vi "set_xwav_attribute_by_name.vi"(8 "Error in":errorcluster caption="Error in (no error)", 9 "value":variant, 10 "name":string, 11 "xwave in":T1={"attributes"=variant, "X"={"start"=0.0, "delta"=0.0, "units"="index", "dim"="au"}, "Y"={"data"=[], "units"="au"}}) -> (0 "Error out":errorcluster, 2 "replaced?":bool, 3 "xwave out":T1={"attributes"=variant, "X"={"start"=0.0, "delta"=0.0, "units"="index", "dim"="au"}, "Y"={"data"=[], "units"="au"}})   [LabVIEW 2015]
uses:
  xwav.ctl
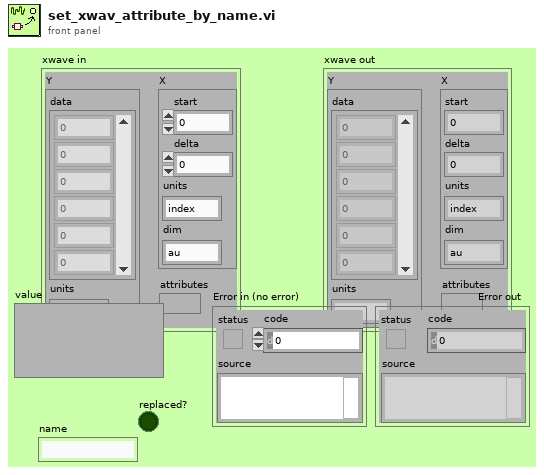
[diagram p1: front panel]
types:
  T1 = typedef "xwav.ctl" = cluster{"attributes":variant, "X":cluster{"start":dbl, "delta":dbl, "units":string, "dim":string}, "Y":cluster{"data":dbl[], "units":string}}
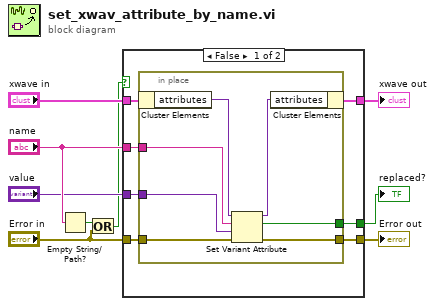
[diagram p0: block diagram]
diagram:
  n1 = Empty String/Path?(string/path="name") -> (empty?=w3:bool)
  n2 = Or(x=w3, y="Error in") -> (x .or. y?=w1:bool)
  n3 = case shown="False" w1 {
    tunnel: "xwave in" -> [w16 w25]
    tunnel: [w15 w25] -> w8
    tunnel: "name" -> [w14 _]
    tunnel: [w13 _] -> w6
    tunnel: "value" -> [w12 _]
    tunnel: "Error in" -> [w11 w24]
    tunnel: [w10 w24] -> w4
    frame False {
      n4 = in-place {
        in-place-border: w14 -> [w21]
        in-place-border: [w20] -> w13
        in-place-border: w12 -> [w19]
        in-place-border: w11 -> [w18]
        in-place-border: [w17] -> w10
        n5 = in-place-cluster #1(w16) -> ("attributes"=w23:variant)
        n6 = Set Variant Attribute(Variant=w23, name=w21, value=w19, error in=w18) -> (Variant out=w22:variant, replaced=w20:bool, error out=w17:errorcluster)
        n7 = in-place-cluster #1("attributes"=w22) -> (w15:T1)
      }
    }
    frame True {
    }
  }
  "xwave out" <- w8
  "replaced?" <- w6
  "Error out" <- w4
